vi "MaxiGauge_Main_Panel.vi"(7 "stop_external":refnum<vi>, 8 "input cluster":T1) -> ()   [LabVIEW 2019]
uses:
  cluster_ref_MaxiGauge.ctl
panel:
  out "status_log":bool caption="Status"
  out "status_read":bool caption="Readout Status"
  in  "Tab Control":enum32{"Ch. 1 & 2", "Ch.  3 & 4", "Ch.  5 & 6"}(tab)
  out "Ch. 1 Chart":waveform(dbl)[](graph)
  out "Ch. 2 Chart":waveform(dbl)[](graph)
  out "Ch. 3 Chart":waveform(dbl)[](graph)
  out "Ch. 4 Chart":waveform(dbl)[](graph)
  out "Ch. 5 Chart":waveform(dbl)[](graph)
  out "Ch. 6 Chart":waveform(dbl)[](graph)
  in  "Logging":bool=TRUE
  out "Ch. 6":dbl
  out "Ch. 5":dbl
  out "Ch. 4":dbl
  out "Ch. 3":dbl
  out "Ch. 2":dbl
  out "Ch. 1":dbl
  in  "stop":bool
  out "Last Measurement":timestamp format="%<%Y-%m-%d %H:%M:%S>T"
  out "GAUGE  Status":string caption="(Channel 1, 2, 3, 4, 5, 6)"
  in  "Channel 6":enum16{"NO CHANGE", "OFF", "ON"}(ring)
  in  "Channel 5":enum16{"NO CHANGE", "OFF", "ON"}(ring)
  in  "Channel 4":enum16{"NO CHANGE", "OFF", "ON"}(ring)
  in  "Channel 3":enum16{"NO CHANGE", "OFF", "ON"}(ring)
  in  "Channel 2":enum16{"NO CHANGE", "OFF", "ON"}(ring)
  in  "Channel 1":enum16{"NO CHANGE", "OFF", "ON"}(ring)
  in  "Change gauge status":bool
  out "Sensor Type":string caption="(Channel 1, 2, 3, 4, 5, 6)"
  in  "Check Sensor Type":bool
  in  "VISA":refnum<visa-resource-name>="COM8"
  in  "Measurement Rate (ms)":i32=5000
  # "MaxiGauge Panel"
  # "Gauge On/Off/Status"
  # "Pressure Value (Torr)"
  # "Torr"
  # "1 = OFF\n2 = ON"
  # "Chart-Axis Control"
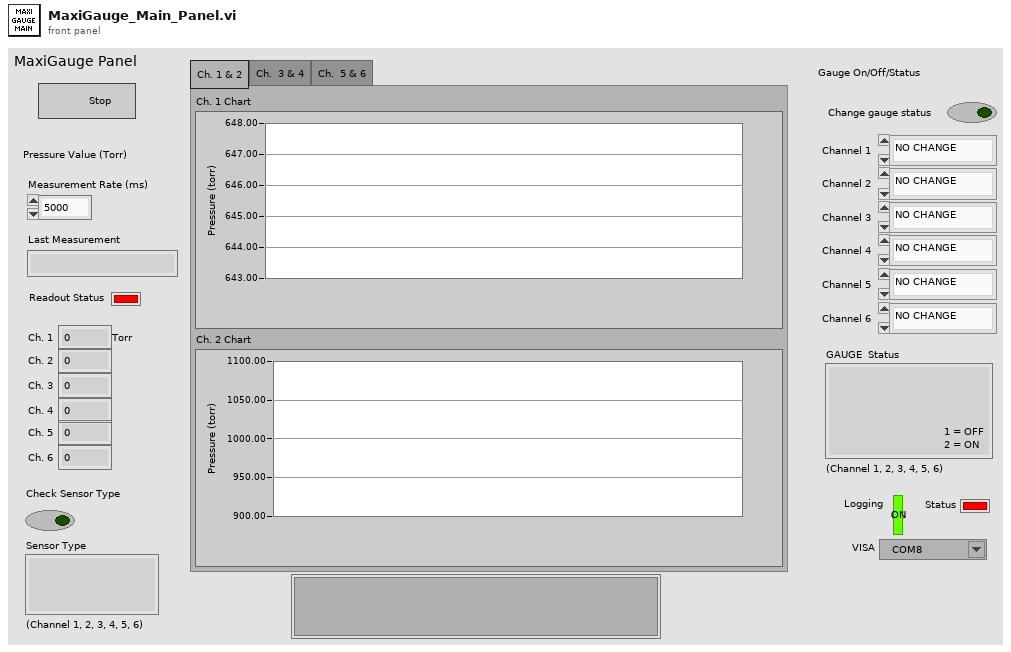
[diagram p1: front panel]
types:
  T1 = typedef "cluster_ref_MaxiGauge.ctl" = cluster{"status":refnum<vi>, "MG1":refnum<vi>, "MG2":refnum<vi>, "MG3":refnum<vi>, "MG4":refnum<vi>}
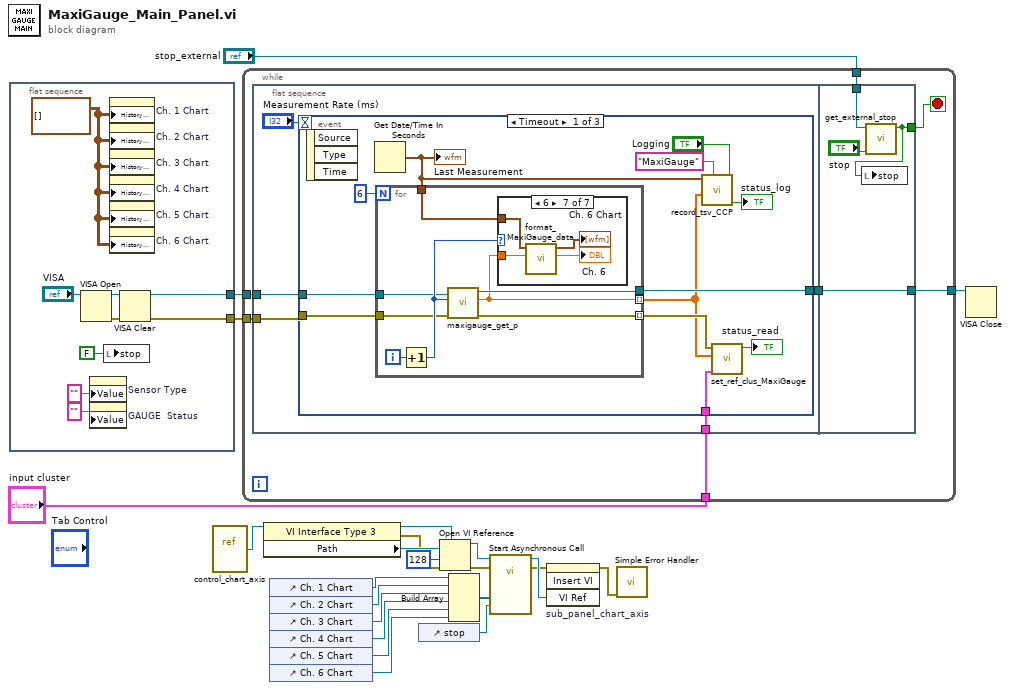
[diagram p0: block diagram]
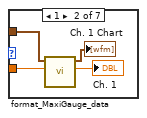
[diagram p3: hidden frame]
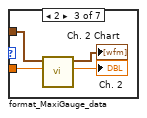
[diagram p4: hidden frame]
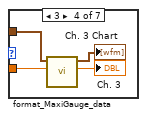
[diagram p5: hidden frame]
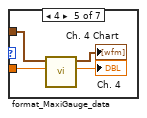
[diagram p6: hidden frame]
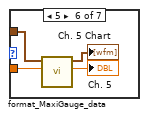
[diagram p7: hidden frame]
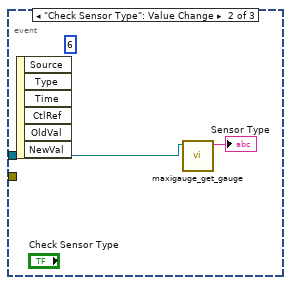
[diagram p8: hidden frame]
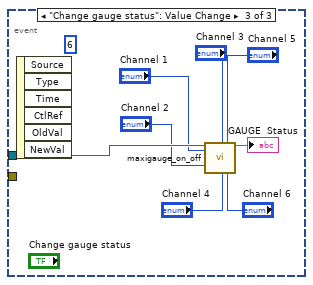
[diagram p9: hidden frame]
diagram:
  n1 = flat-sequence {
    tunnel: [w30] -> w21
    tunnel: [w28] -> w20
    frame #0 {
      w25 = waveform(dbl)[][] [] ("History Data")
      n2 = VISA Open(VISA resource name="VISA") -> (VISA resource name=w32:refnum<visa-resource-name>, error out=w29:errorcluster)  [unwired: 4 in]
      n3 = property on="Sensor Type" class="Str"("Value"="" ("Sensor Type")) -> ()  [unwired: 2 in, 2 out]
      n4 = property on="GAUGE  Status" class="Str"("Value"="" ("GAUGE  Status")) -> ()  [unwired: 2 in, 2 out]
      n5 = local write "stop"(FALSE ("stop")) -> ()
      n6 = property on="Ch. 1 Chart" class="WFChart (strict)"("History Data"=w25) -> ()  [unwired: 2 in, 2 out]
      n7 = property on="Ch. 2 Chart" class="WFChart (strict)"("History Data"=w25) -> ()  [unwired: 2 in, 2 out]
      n8 = property on="Ch. 3 Chart" class="WFChart (strict)"("History Data"=w25) -> ()  [unwired: 2 in, 2 out]
      n9 = property on="Ch. 4 Chart" class="WFChart (strict)"("History Data"=w25) -> ()  [unwired: 2 in, 2 out]
      n10 = property on="Ch. 5 Chart" class="WFChart (strict)"("History Data"=w25) -> ()  [unwired: 2 in, 2 out]
      n11 = property on="Ch. 6 Chart" class="WFChart (strict)"("History Data"=w25) -> ()  [unwired: 2 in, 2 out]
      n12 = VISA Clear(VISA resource name=w32, error in (no error)=w29) -> (VISA resource name out=w30:refnum<visa-resource-name>, error out=w28:errorcluster)
    }
  }
  n13 = vi-ref "control_chart_axis.vi"() -> (w17:refnum<vi>)
  n14 = while {
    tunnel: "input cluster" -> [w39]
    tunnel: w21 -> [w38]
    tunnel: [w37] -> w22
    tunnel: w20 -> [w36]
    tunnel: "stop_external" -> [w34]
    stop <- w33 stop-if-true
    n15 = flat-sequence {
      tunnel: w39 -> [w43]
      tunnel: w38 -> [w42]
      tunnel: w36 -> [w40]
      tunnel: [w41] -> w35
      tunnel: [w102] -> w37
      tunnel: w35 -> [w102]
      tunnel: w34 -> [w100]
      tunnel: [w99] -> w33
      frame #0 {
        n16 = event shown="[0] Timeout" {
          selector: _ -> [_ _ _]
          dyn-events: _ -> [_ _ _]
          timeout: "Measurement Rate (ms)" -> [_ _ _]
          tunnel: w42 -> [w55 w90 w98]
          tunnel: w43 -> [w54 _ _]
          tunnel: [w52 _ _] -> w41
          tunnel: w40 -> [w51 _ _]
          event Timeout {
            n17 = event-data() -> ()  [unwired: 1 in, 3 out]
            n18 = Get Date/Time In Seconds() -> (seconds since 1Jan1904=w48:timestamp)
            "Last Measurement" <- w48
            n19 = for {
              N: 6 -> [_]
              tunnel: w55 -> [w62]
              tunnel: [w58] -> w47 mode=indexing
              tunnel: [w61] -> w53 mode=indexing
              tunnel: [w60] -> w52
              tunnel: w51 -> [w59]
              tunnel: w48 -> [w57]
              i -> [w64]
              n20 = Increment(x=w64) -> (x+1=w63:i32)
              n21 = call "maxigauge_get_p.vi"("err_in"=w59, "sensor_number"=w63, "visa_in"=w62) -> ("err_out"=w61:errorcluster, "pressure"=w58:dbl, "visa_out"=w60:refnum<visa-resource-name>)  [unwired: 5 in, 1 out]
              n22 = case shown="6" w63 {
                tunnel: w58 -> [_ w68 w72 w75 w79 w84 w87]
                tunnel: w57 -> [_ w65 w70 w74 w78 w81 w85]
                frame 0, Default {
                }
                frame 1 {
                  n23 = call "format_MaxiGauge_data.vi"("pressure"=w68, "time"=w65) -> ("pressure_out"=→"Ch. 1":dbl, "waveform_array"=→"Ch. 1 Chart":waveform(dbl)[])  [unwired: 8 in]
                }
                frame 2 {
                  n24 = call "format_MaxiGauge_data.vi"("pressure"=w72, "time"=w70) -> ("pressure_out"=→"Ch. 2":dbl, "waveform_array"=→"Ch. 2 Chart":waveform(dbl)[])  [unwired: 8 in]
                }
                frame 3 {
                  n25 = call "format_MaxiGauge_data.vi"("pressure"=w75, "time"=w74) -> ("pressure_out"=→"Ch. 3":dbl, "waveform_array"=→"Ch. 3 Chart":waveform(dbl)[])  [unwired: 8 in]
                }
                frame 4 {
                  n26 = call "format_MaxiGauge_data.vi"("pressure"=w79, "time"=w78) -> ("pressure_out"=→"Ch. 4":dbl, "waveform_array"=→"Ch. 4 Chart":waveform(dbl)[])  [unwired: 8 in]
                }
                frame 5 {
                  n27 = call "format_MaxiGauge_data.vi"("pressure"=w84, "time"=w81) -> ("pressure_out"=→"Ch. 5":dbl, "waveform_array"=→"Ch. 5 Chart":waveform(dbl)[])  [unwired: 8 in]
                }
                frame 6 {
                  n28 = call "format_MaxiGauge_data.vi"("pressure"=w87, "time"=w85) -> ("pressure_out"=→"Ch. 6":dbl, "waveform_array"=→"Ch. 6 Chart":waveform(dbl)[])  [unwired: 8 in]
                }
              }
            }
            n29 = call "record_tsv_CCP.vi"("logging_on"="Logging", "folder_name"="MaxiGauge", "value_array"=w47, "time"=w48) -> ("status"=→"status_log":bool)  [unwired: 6 in, 1 out]
            n30 = call "set_ref_clus_MaxiGauge.vi"("input cluster"=w54, "value_array"=w47, "error_array"=w53) -> ("status"=→"status_read":bool)  [unwired: 8 in]
          }
          event "Check Sensor Type": Value Change {
            (unwired) 6
            n31 = event-data() -> ()  [unwired: 1 in, 6 out]
            n32 = call "maxigauge_get_gauge.vi"("maxi_visa"=w90) -> ("Gauge Type"=→"Sensor Type":string)  [unwired: 8 in, 1 out]
          }
          event "Change gauge status": Value Change {
            (unwired) 6
            n33 = event-data() -> ()  [unwired: 1 in, 6 out]
            n34 = call "maxigauge_on_off.vi"("VISA"=w98, "Channel 1"="Channel 1", "Channel 2"="Channel 2", "Channel 3"="Channel 3", "Channel 4"="Channel 4", "Channel 5"="Channel 5", "Channel 6"="Channel 6") -> ("string"=→"GAUGE  Status":string)  [unwired: 11 in, 1 out]
          }
        }
      }
      frame #1 {
        n35 = call "get_external_stop.vi"("stop_internal"="stop", "ref_stop_external"=w100) -> ("stop_output"=w99:bool)  [unwired: 9 in]
        n36 = local write "stop"(w99) -> ()
      }
    }
  }
  n37 = property class="VI Interface Type 3"(reference=w17) -> (reference out=w15:refnum<vi>, error out=w14:errorcluster, "Path"=w18:path)  [unwired: 1 in]
  n38 = control-ref of="Ch. 1 Chart"() -> (w6:refnum<vi>)
  n39 = control-ref of="Ch. 2 Chart"() -> (w5:refnum<vi>)
  n40 = control-ref of="Ch. 3 Chart"() -> (w4:refnum<vi>)
  n41 = control-ref of="Ch. 4 Chart"() -> (w3:refnum<vi>)
  n42 = control-ref of="Ch. 5 Chart"() -> (w2:refnum<vi>)
  n43 = control-ref of="Ch. 6 Chart"() -> (w1:refnum<vi>)
  n44 = control-ref of="stop"() -> (w8:refnum<vi>)
  n45 = Open VI Reference(type specifier VI Refnum (for type only)=w15, vi path=w18, options=128, error in (no error)=w14) -> (vi reference=w9:refnum<vi>, error out=w10:errorcluster)  [unwired: 2 in]
  n46 = Build Array(w6, w5, w4, w3, w2, w1) -> (w7:refnum<vi>[])
  n47 = call-by-ref "Start Asynchronous Call"(reference=w9, error in=w10, "stop"=w8, "chart_array"=w7) -> (reference out=w13:refnum<vi>, error out=w12:errorcluster)  [unwired: 10 in]
  n48 = invoke on="sub_panel_chart_axis" class="SubPnl" method="Insert VI"(error in=w12, "VI Ref"=w13) -> (error out=w11:errorcluster)  [unwired: 2 in, 3 out]
  n49 = call <vilib>:"Simple Error Handler.vi"("error in (no error)"=w11) -> ()  [unwired: 4 in, 5 out]
  n50 = VISA Close(VISA resource name=w22) -> ()  [unwired: 1 in, 1 out]
